vi "Run.vi"(8 "error in (no error)":errorcluster caption="entrée d'erreur (pas d'erreur)", 11 "Johnson_lindenstrauss_min_dim.lvclass":refnum<class "Johnson_lindenstrauss_min_dim.lvclass">) -> (0 "error out":errorcluster caption="sortie d'erreur", 2 "Data":T1, 3 "Johnson_lindenstrauss_min_dim.lvclass":refnum<class "Johnson_lindenstrauss_min_dim.lvclass">)   [LabVIEW 2020, in "Johnson_lindenstrauss_min_dim.lvclass"]
doc: "Find a ‘safe’ number of components to randomly project to\n\nThe distortion introduced by a random projection p only changes the distance between two points by a factor (1 +- eps) in an euclidean space with good probability. The projection p is an eps-embedding as defined by:\n\n(1 - eps) ||u - v||^2 < ||p(u) - p(v)||^2 < (1 + eps) ||u - v||^2\n\nWhere u and v are any rows taken from a dataset of shape [n_samples, n_features], eps is in ]0, 1[ and p is a projection by a random Gaussian N(0, 1) matrix with shape [n_components, n_features] (or a sparse Achlioptas matrix).\n\nThe minimum number of components to guarantee the eps-embedding is given by:\n\nn_components >= 4 log(n_samples) / (eps^2 / 2 - eps^3 / 3)\n\nNote that the number of dimensions is independent of the original number of features but instead depends on the size of the dataset: the larger the dataset, the higher is the minimal dimensionality of an eps-embedding.\n\n\nReturns : \n\n- n_components : int or numpy array of int,\nThe minimal number of components to guarantee with good probability an eps-embedding with n_samples."
uses:
  Johnson_lindenstrauss_min_dim.lvclass
  Johnson_lindenstrauss_min_dim.lvclass/Johnson_lindenstrauss_min_dim.ctl
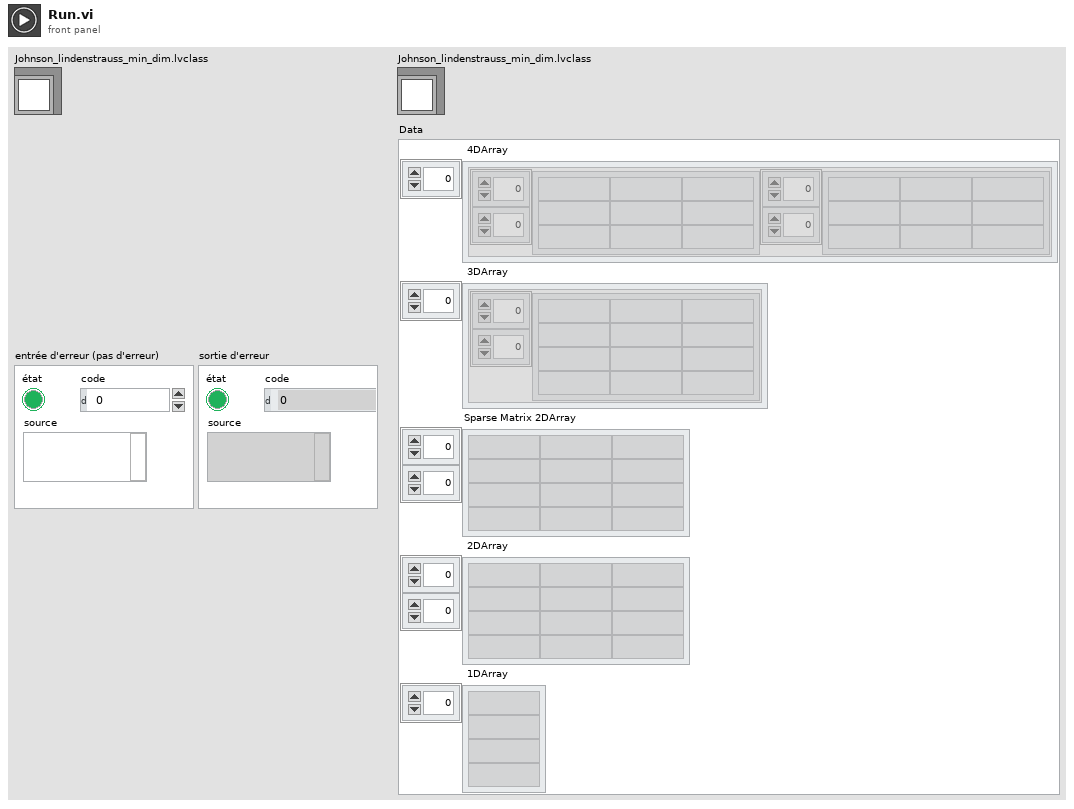
[diagram p1: front panel]
types:
  T1 = cluster{" 4DArray":cluster{"1":string[][], "2":string[][]}[], " 3DArray":cluster{"Tableau":string[][]}[], "Sparse Matrix 2DArray":string[][], " 2DArray":string[][], " 1DArray":string[]}
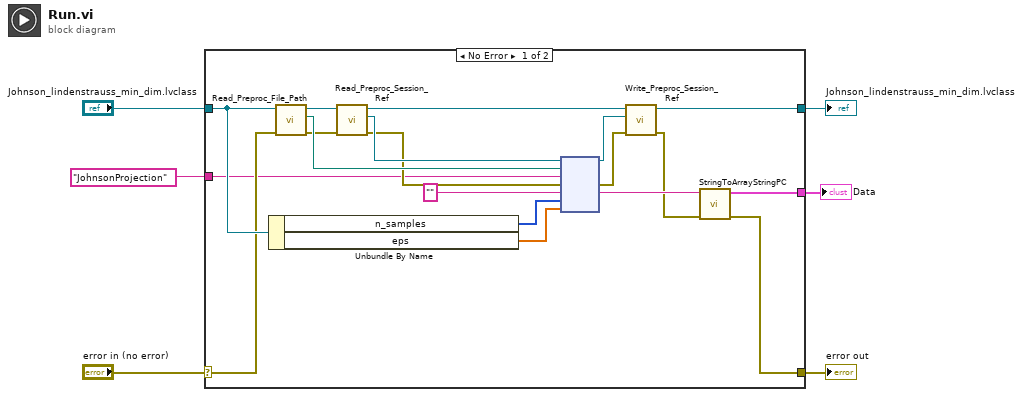
[diagram p0: block diagram]
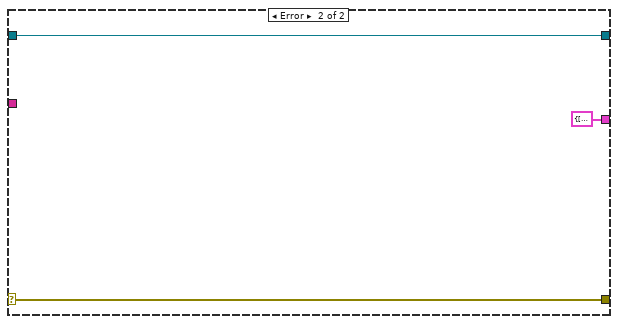
[diagram p2: hidden frame]
diagram:
  n1 = case shown="No Error" "error in (no error)" {
    selector: "error in (no error)" -> [w15 w28]
    tunnel: [w8 w28] -> w5
    tunnel: [w10 w27] -> w3
    tunnel: "Johnson_lindenstrauss_min_dim.lvclass" -> [w16 w27]
    tunnel: "JohnsonProjection" ("Fonction") -> [w14 _]
    tunnel: [w7 T1 {" 4DArray"=[], " 3DArray"=[], "Sparse Matrix 2DArray"=[], " 2DArray"=[], " 1DArray"=[]} ("Data")] -> w1
    frame No Error {
      n2 = Unbundle By Name(w16) -> ("n_samples"=w13:i32[], "eps"=w12:dbl[])
      n3 = call-dynamic "Read_Preproc_File_Path.vi"("error in (no error)"=w15, "Python in"=w16) -> ("error out"=w20:errorcluster, "File_Path"=w23:path, "Python out"=w25:refnum<class "Johnson_lindenstrauss_min_dim.lvclass">)  [unwired: 7 in]
      n4 = call-dynamic "Read_Preproc_Session_Ref.vi"("error in (no error)"=w20, "Python in"=w25) -> ("error out"=w21:errorcluster, "Session_ref"=w22:refnum<k35>, "Python out"=w24:refnum<class "Johnson_lindenstrauss_min_dim.lvclass">)  [unwired: 7 in]
      n5 = node(w22, w23, w14, w21, "", w13, w12) -> (w17:refnum<k35>, w19:errorcluster, w11:string)  [unwired: 2 in, 2 out]
      n6 = call-dynamic "Write_Preproc_Session_Ref.vi"("error in (no error)"=w19, "Session_ref"=w17, "Python in"=w24) -> ("error out"=w9:errorcluster, "Python out"=w10:refnum<class "Johnson_lindenstrauss_min_dim.lvclass">)  [unwired: 7 in]
      n7 = call "StringToArrayStringPC.vi"("sortie d'erreur"=w9, "Return value"=w11) -> ("sortie d'erreur"=w8:errorcluster, "Data"=w7:T1)  [unwired: 8 in]
    }
    frame Error {
    }
  }
  "error out" <- w5
  "Johnson_lindenstrauss_min_dim.lvclass" <- w3
  "Data" <- w1
